vi "CAlex_ChangeDate.vi"() -> ()   [LabVIEW 2015]
uses:
  CustomVIs/CustomVI.lvlib
panel:
  in  "Multicolumn Listbox":i32(listbox)
  in  "Path":path
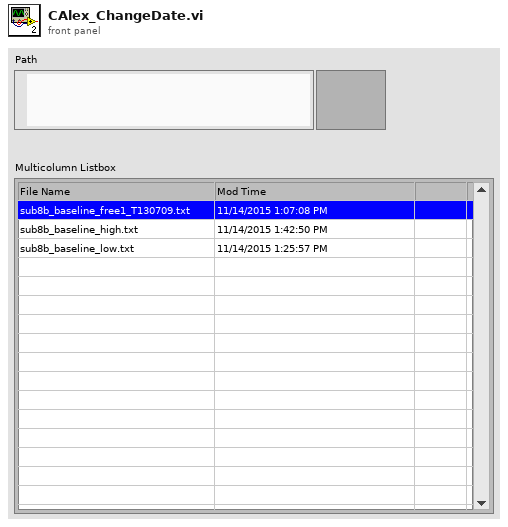
[diagram p1: front panel]
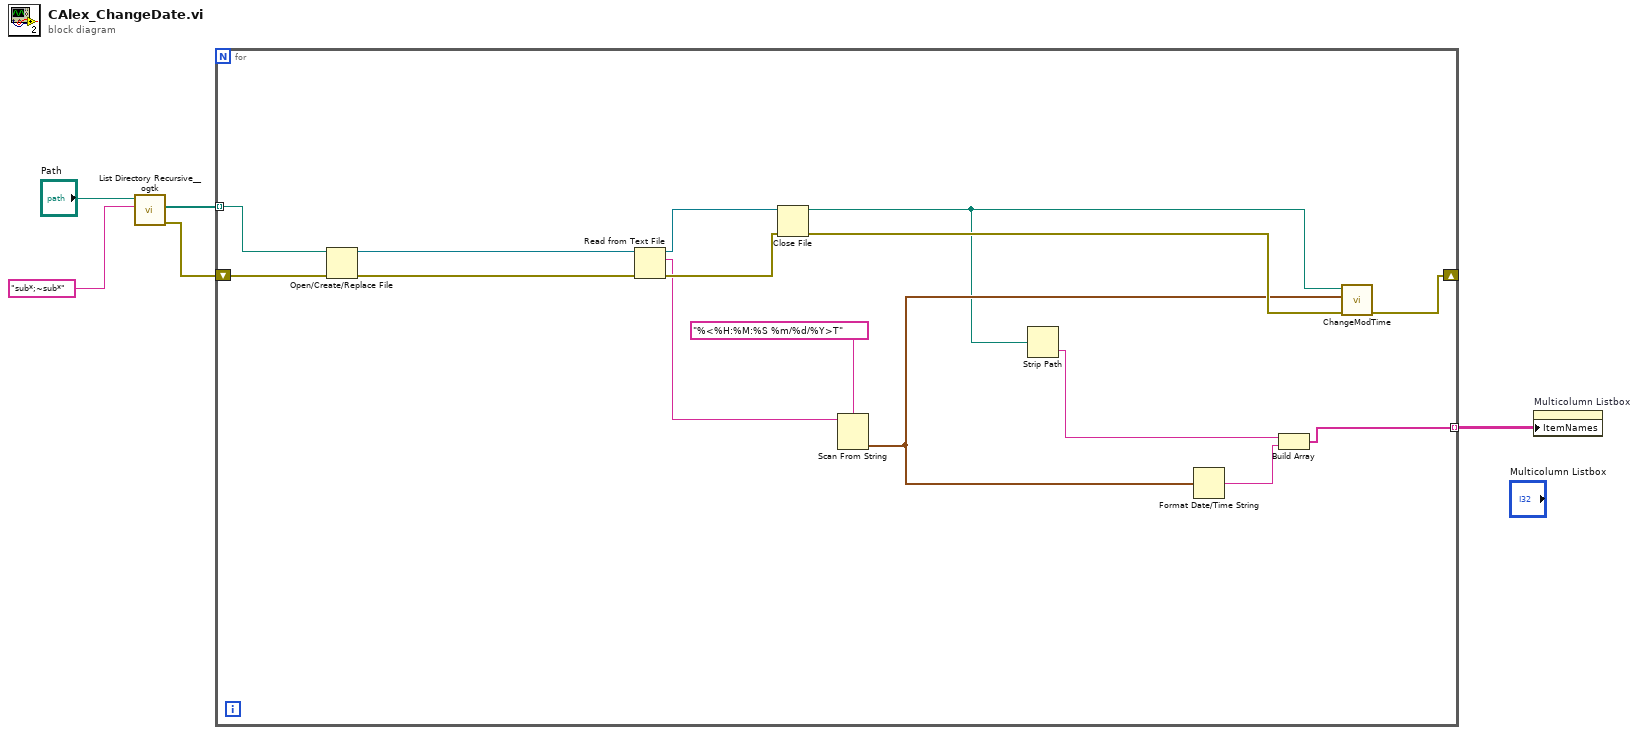
[diagram p0: block diagram]
diagram:
  n1 = call <userlib>:"List Directory Recursive__ogtk.vi"("pattern"="sub*;~sub*", "Path"="Path") -> ("error out"=w4:errorcluster, "file paths"=w2:path[])  [unwired: 6 in, 2 out]
  n2 = for {
    shift-right: [w15] -> _
    shift-left: w4 -> [w16]
    tunnel: w2 -> [w12] mode=indexing
    tunnel: [w8] -> w1 mode=indexing
    n3 = Open/Create/Replace File(file path (use dialog)=w12, error in=w16) -> (refnum out=w14:refnum<file>, error out=w13:errorcluster)  [unwired: 4 in, 1 out]
    n4 = Read from Text File(file (use dialog)=w14, error in=w13) -> (refnum out=w19:refnum<file>, text=w10:string, error out=w20:errorcluster)  [unwired: 2 in, 1 out]
    n5 = Close File(refnum=w19, error in=w20) -> (path=w7:path, error out=w18:errorcluster)
    n6 = Scan From String(format string="%<%H:%M:%S %m/%d/%Y>T", input string=w10) -> (output 1=w11:timestamp)  [unwired: 3 in, 3 out]
    n7 = Strip Path(path=w7) -> (name=w6:string)  [unwired: 1 out]
    n8 = Format Date/Time String(seconds (now)=w11) -> (date/time string=w9:string)  [unwired: 2 in]
    n9 = Build Array(w6, w9) -> (w8:string[])
    n10 = call "ChangeModTime.vi"("error in (no error)"=w18, "Time Stamp"=w11, "path"=w7) -> ("error out"=w15:errorcluster)  [unwired: 7 in, 1 out]
  }
  n11 = property on="Multicolumn Listbox" class="MCListbox (strict)"("ItemNames"=w1) -> ()  [unwired: 2 in, 2 out]
